vi "instance count allowed.vi"(8 "error in":errorcluster, 11 "engine configuration in":refnum<class "base TBM sequencer configuration.lvclass">) -> (0 "error out":errorcluster, 2 "instances allowed (-1 = no limit)":i32, 3 "engine configuration out":refnum<class "base TBM sequencer configuration.lvclass">)   [LabVIEW 2014, in "base TBM sequencer configuration.lvclass"]
doc: "This property is used to specify how many instances of a particular type of engine are allowed in memory on a target at the same time."
uses:
  base TBM sequencer configuration.lvclass
  <vilib>/NI/Tag Bus Module Framework/module configuration/TBM module configuration.lvclass
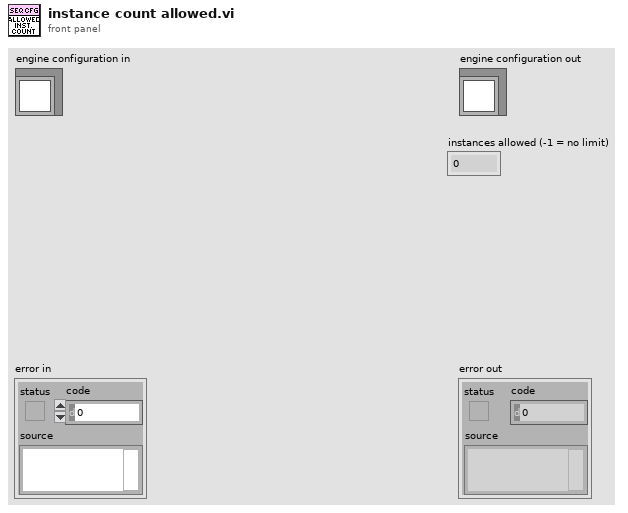
[diagram p1: front panel]
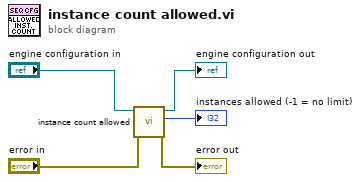
[diagram p0: block diagram]
diagram:
  n1 = call-parent "instance count allowed.vi"("error in"="error in", "module configuration in"="engine configuration in") -> ("error out"=→"error out":errorcluster, "instances allowed"=→"instances allowed (-1 = no limit)":i32, "module configuration out"=→"engine configuration out":refnum<class "base TBM sequencer configuration.lvclass">)  [unwired: 7 in]
